vi "Galil_address.vi"() -> ()   [LabVIEW 2010]
panel:
  in  "Galil.IGalil":refnum<k7>
  out "Library Version:":string
  out "error out":errorcluster
  out "Connected To:":string
  in  "Connection String:":string
  # "This vi Shows how to use the address member of the Galil Communications Library.  \n\nIf Connection String is left blank, the vi will open the connections dialog when run.  If a value is input into Connection String, the vi will attempt to connect to the controller at that address (ex COM1 19200)."
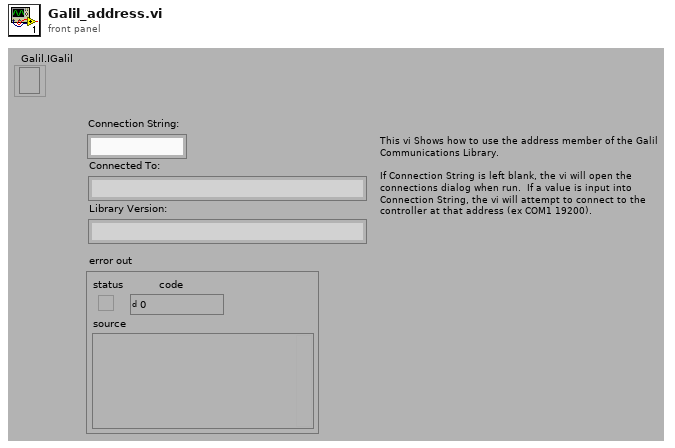
[diagram p1: front panel]
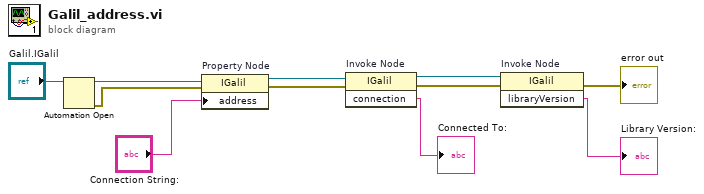
[diagram p0: block diagram]
diagram:
  n1 = Automation Open(Automation Refnum="Galil.IGalil") -> (Automation Refnum=w11:refnum<k7>, error out=w9:errorcluster)  [unwired: 1 in, 2 out]
  n2 = property on="Property Node" class="IGalil"(reference=w11, error in=w9, "address"="Connection String:") -> (reference out=w10:refnum<k7>, error out=w8:errorcluster)
  n3 = invoke on="Invoke Node" class="IGalil" method="connection"(reference=w10, error in=w8) -> (reference out=w5:refnum<k7>, error out=w4:errorcluster, "connection"=→"Connected To:":string)  [unwired: 1 in]
  n4 = invoke on="Invoke Node" class="IGalil" method="libraryVersion"(reference=w5, error in=w4) -> (error out=→"error out":errorcluster, "libraryVersion"=→"Library Version:":string)  [unwired: 1 in, 1 out]
